vi "Attitude Control Write.vi"(8 "error in (no error)":errorcluster, 10 "pitch (x), roll (y), yaw (z)":T2, 11 "Attitude Control Handle In":T1) -> (0 "error out":errorcluster, 3 "Attitude Control Handle Out":T1)   [LabVIEW 2015, in "RDS Libraries.lvlib" / "lv-attitudecontrol.lvlib"]
uses:
  lv-attitudecontrol.lvlib
  <vilib>/Utility/miscctls.llb/LV3DPointTypeDef.ctl
  Controls/AttitudeHandle.ctl
  <vilib>/picture/3D Picture Control/NI_3D Picture Control.lvlib
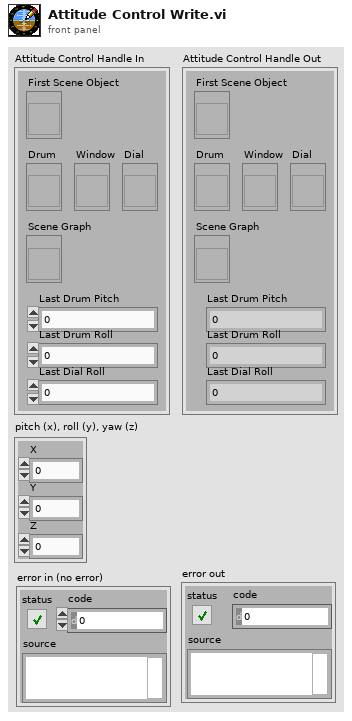
[diagram p1: front panel]
types:
  T1 = typedef "RDS Libraries.lvlib/lv-attitudecontrol.lvlib/AttitudeHandle.ctl" = cluster{"First Scene Object":refnum<vi>, "Drum":refnum<vi>, "Window":refnum<vi>, "Dial":refnum<vi>, "Scene Graph":refnum<vi>, "Last Drum Pitch":dbl, "Last Drum Roll ":dbl, "Last Dial Roll":dbl}
  T2 = typedef "LV3DPointTypeDef.ctl" = cluster{"X":sgl, "Y":sgl, "Z":sgl}
  T3 = enum16{"None", "Spherical", "Flying", "Oriented"}
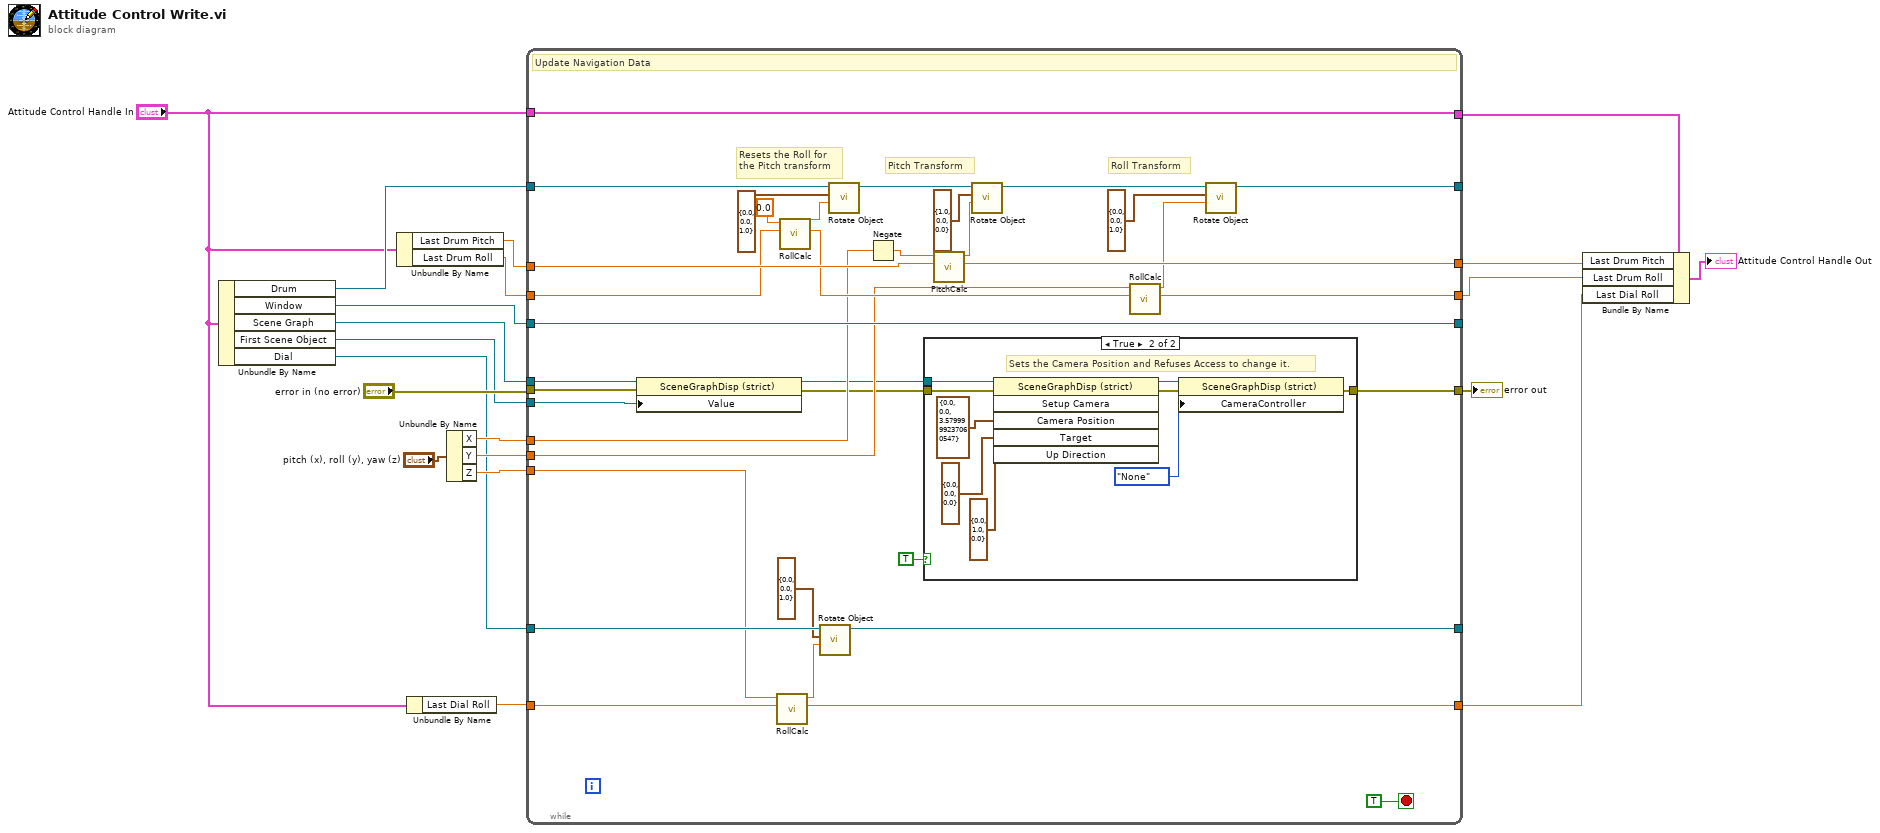
[diagram p0: block diagram]
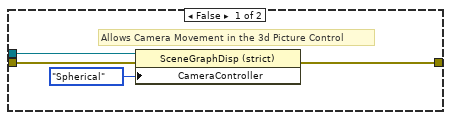
[diagram p2: hidden frame]
diagram:
  n1 = Unbundle By Name("Attitude Control Handle In") -> ("Drum"=w14:refnum<vi>, "Window"=w15:refnum<vi>, "Scene Graph"=w9:refnum<vi>, "First Scene Object"=w8:refnum<vi>, "Dial"=w7:refnum<vi>)
  n2 = Unbundle By Name("Attitude Control Handle In") -> ("Last Drum Pitch"=w12:dbl, "Last Drum Roll"=w11:dbl)
  n3 = Unbundle By Name("Attitude Control Handle In") -> ("Last Dial Roll"=w10:dbl)
  n4 = Unbundle By Name("pitch (x), roll (y), yaw (z)") -> ("X"=w18:sgl, "Y"=w19:sgl, "Z"=w20:sgl)
  n5 = while {
    tunnel: w15 -> [w54]
    tunnel: w14 -> [w56]
    tunnel: [w54] -> _
    tunnel: [w53] -> _
    tunnel: w7 -> [w46]
    tunnel: [w44] -> _
    tunnel: "error in (no error)" -> [w27]
    tunnel: [w33] -> w13
    tunnel: w18 -> [w30]
    tunnel: w19 -> [w29]
    tunnel: w20 -> [w28]
    tunnel: w9 -> [w22]
    tunnel: w8 -> [w26]
    tunnel: "Attitude Control Handle In" -> [w21]
    tunnel: [w21] -> w4
    tunnel: w12 -> [w51]
    tunnel: [w50] -> w3
    tunnel: w11 -> [w48]
    tunnel: [w52] -> w2
    tunnel: w10 -> [w47]
    tunnel: [w45] -> w1
    stop <- TRUE stop-if-true
    # "Roll Transform"
    # "Resets the Roll for \nthe Pitch transform"
    # "Pitch Transform"
    # "Update Navigation Data"
    n6 = property on="Property Node" class="SceneGraphDisp (strict)"(reference=w22, error in=w27, "Value"=w26) -> (reference out=w24:refnum<vi>, error out=w25:errorcluster)
    n7 = call "RollCalc.vi"("Previous Roll Value"=w47, "Roll Input"=w28) -> ("New Roll Value"=w45:dbl, "Adjustment to be Made"=w43:dbl)  [unwired: 8 in]
    n8 = call "RollCalc.vi"("Previous Roll Value"=w48, "Roll Input"=sgl 0.0 ("Angle")) -> ("New Roll Value"=w49:dbl, "Adjustment to be Made"=w38:dbl)  [unwired: 8 in]
    n9 = call <vilib>:"Rotate Object.vi"("Angle"=w43, "Axis"=cluster{"X":sgl, "Y":sgl, "Z":sgl} {"X"=0.0, "Y"=0.0, "Z"=1.0} ("Axis 2"), "Scene.Object In"=w46) -> ("Scene.Object Out"=w44:refnum<vi>)  [unwired: 7 in, 1 out]
    n10 = call <vilib>:"Rotate Object.vi"("Angle"=w38, "Axis"=cluster{"X":sgl, "Y":sgl, "Z":sgl} {"X"=0.0, "Y"=0.0, "Z"=1.0} ("Axis 2"), "Scene.Object In"=w56) -> ("Scene.Object Out"=w39:refnum<vi>)  [unwired: 7 in, 1 out]
    n11 = Negate(x=w30) -> (-x=w31:sgl)
    n12 = case shown="True" TRUE {
      tunnel: [w58 w63] -> w33
      tunnel: w25 -> [w60 w65]
      tunnel: w24 -> [w57 w62]
      frame False {
        # "Allows Camera Movement in the 3d Picture Control"
        n13 = property on="Property Node" class="SceneGraphDisp (strict)"(reference=w57, error in=w60, "CameraController"=T3."Spherical" ("Camera Controller:Type")) -> (error out=w58:errorcluster)  [unwired: 1 out]
      }
      frame True {
        # "Sets the Camera Position and Refuses Access to change it."
        n14 = invoke on="Invoke Node" class="SceneGraphDisp (strict)" method="Setup Camera"(reference=w62, error in=w65, "Camera Position"=T2 {"X"=0.0, "Y"=0.0, "Z"=3.58}, "Target"=T2 {"X"=0.0, "Y"=0.0, "Z"=0.0}, "Up Direction"=T2 {"X"=0.0, "Y"=1.0, "Z"=0.0}) -> (reference out=w61:refnum<vi>, error out=w64:errorcluster)  [unwired: 1 in, 4 out]
        n15 = property on="Property Node" class="SceneGraphDisp (strict)"(reference=w61, error in=w64, "CameraController"=T3."None" ("Camera Controller:Type")) -> (error out=w63:errorcluster)  [unwired: 1 out]
      }
    }
    n16 = call "PitchCalc.vi"("Previous Pitch Value"=w51, "Pitch Control"=w31) -> ("New Pitch Value"=w50:dbl, "Adjustment to be made"=w40:dbl)  [unwired: 8 in]
    n17 = call <vilib>:"Rotate Object.vi"("Angle"=w40, "Axis"=cluster{"X":sgl, "Y":sgl, "Z":sgl} {"X"=1.0, "Y"=0.0, "Z"=0.0} ("Axis 2"), "Scene.Object In"=w39) -> ("Scene.Object Out"=w55:refnum<vi>)  [unwired: 7 in, 1 out]
    n18 = call "RollCalc.vi"("Previous Roll Value"=w49, "Roll Input"=w29) -> ("New Roll Value"=w52:dbl, "Adjustment to be Made"=w34:dbl)  [unwired: 8 in]
    n19 = call <vilib>:"Rotate Object.vi"("Angle"=w34, "Axis"=cluster{"X":sgl, "Y":sgl, "Z":sgl} {"X"=0.0, "Y"=0.0, "Z"=1.0} ("Axis 2"), "Scene.Object In"=w55) -> ("Scene.Object Out"=w53:refnum<vi>)  [unwired: 7 in, 1 out]
  }
  "error out" <- w13
  n20 = Bundle By Name(cluster=w4, "Last Drum Pitch"=w3, "Last Drum Roll"=w2, "Last Dial Roll"=w1) -> (→"Attitude Control Handle Out":T1)
